vi "grabberpidinit.vi"(9 "setpoint":dbl format="%.2f", 11 "reinitialize? (F) 2":bool) -> (0 "Done? 2":bool)   [LabVIEW 2013]
uses:
  <vilib>/addons/control/pid/pid.llb/PID (DBL).vi
  <vilib>/addons/control/pid/NI_PID_pid.lvlib
panel:
  in  "adjuster":dbl
  in  "PID Gains for Raising/Lowering":T1={"proportional gain (Kc)"=1.2, "integral time (Ti, min)"=0.011, "derivative time (Td, min)"=0.007} {"derivative time (Td, min)" format="%.3f"; "integral time (Ti, min)" format="%.3f"; "proportional gain (Kc)" format="%.3f"}
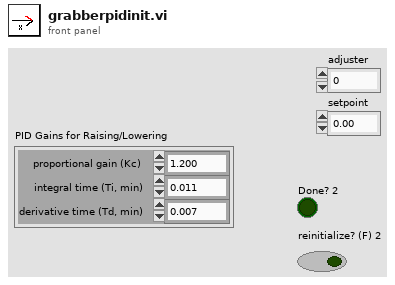
[diagram p1: front panel]
types:
  T1 = cluster{"proportional gain (Kc)":dbl, "integral time (Ti, min)":dbl, "derivative time (Td, min)":dbl}
  T2 = typedef "WPI_EncoderDevRef.ctl" = cluster{"DevStatus":errorcluster, "EncoderIndex":T3, "CounterIndex":T4, "DistancePerCount":dbl, "Decoding Type":T5}
  T3 = typedef "FPGA_EncoderIdx.ctl" = enum8{"Enc 0", "Enc 1", "Enc 2", "Enc 3", "Invalid"}
  T4 = typedef "FPGA_CounterCtrSystemIndex.ctl" = enum8{"Ctr 0", "Ctr 1", "Ctr 2", "Ctr 3", "Ctr 4", "Ctr 5", "Ctr 6", "Ctr 7", "Invalid"}
  T5 = typedef "WPI_EncoderType.ctl" = enum16{"1x", "2x", "4x"}
  T6 = typedef "WPI_MotorControlDeviceRef.ctl" = cluster{"DeviceStatus":errorcluster, "Type":enum16{"PWM", "CAN"}, "PWM":cluster{"Digital Module":T7, "PWM Channel":T8, "DeadBand":T9}, "CAN":cluster{"Device Number":u8, "Control Mode":T10, "Semaphore":T11, "Max Vout":dbl}, "Invert":bool, "TransformRef":T12, "InvTransformRef":T12}
  T7 = typedef "FPGA_TypedefDigitalModule.ctl" = enum16{"Digital Module 1", "Digital Module 2"}
  T8 = typedef "FPGA_DIOPWMChannel.ctl" = enum8{"PWM 1", "PWM 2", "PWM 3", "PWM 4", "PWM 5", "PWM 6", "PWM 7", "PWM 8", "PWM 9", "PWM 10", "Invalid"}
  T9 = typedef "WPI_PWMDeadband.ctl" = cluster{"Name":string, "maxPositivePwm":i32, "minPositivePwm":i32, "centerPwm":i32, "maxNegativePwm":i32, "minNegativePwm":i32, "angularRange":u16}
  T10 = typedef "WPI_CANJaguar_ControlMode.ctl" = enum8{"Percent VBus", "Current", "Speed", "Position", "Voltage"}
  T11 = typedef "Semaphore RefNum" = refnum<k1>
  T12 = typedef "WPI_PWMTransform_ConPane.ctl" = refnum<vi>
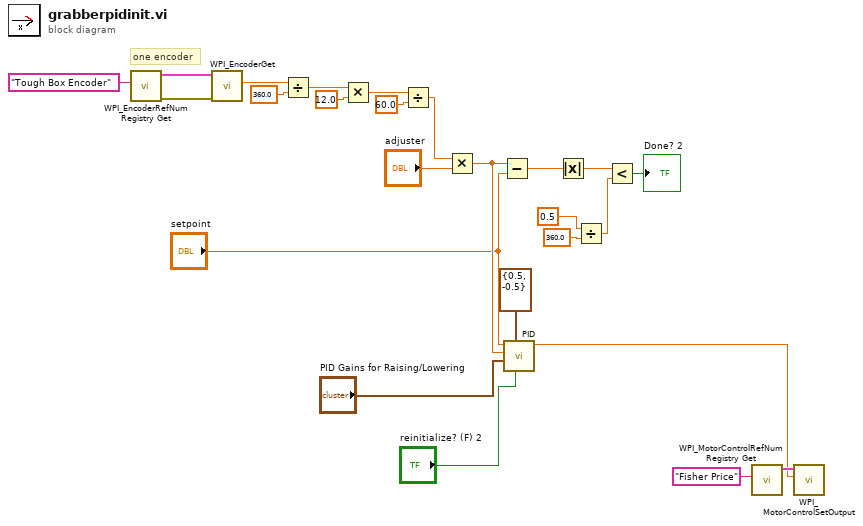
[diagram p0: block diagram]
diagram:
  # "one encoder"
  n1 = call <vilib>:"WPI_EncoderRefNum Registry Get.vi"("refnum name"="Tough Box Encoder") -> ("error out"=w25:errorcluster, "EncoderDevRef"=w24:T2)  [unwired: 9 in]
  n2 = call <vilib>:"WPI_EncoderGet.vi"("error in (no error)"=w25, "EncoderDevRef"=w24) -> ("Distance"=w15:dbl)  [unwired: 4 in, 5 out]
  n3 = Divide(x=w15, y=360.0) -> (x/y=w13:dbl)
  n4 = Multiply(x=w13, y=12.0) -> (x*y=w14:dbl)
  n5 = Divide(x=w14, y=60.0) -> (x/y=w10:dbl)
  n6 = Multiply(x=w10, y="adjuster") -> (x*y=w8:dbl)
  n7 = Subtract(x=w8, y="setpoint") -> (x-y=w20:dbl)
  n8 = call-poly <vilib>:"PID.vi"("reinitialize? (F)"="reinitialize? (F) 2", "output range"=cluster{"output high":dbl, "output low":dbl} {"output high"=0.5, "output low"=-0.5}, "PID gains"="PID Gains for Raising/Lowering", "process variable"=w8, "setpoint"="setpoint") -> ("output"=w1:dbl)  [unwired: 5 in, 1 out]
  n9 = Absolute Value(x=w20) -> (abs(x)=w21:dbl)
  n10 = Divide(x=0.5, y=360.0) -> (x/y=w4:dbl)
  n11 = Less?(x=w21, y=w4) -> (x < y?=→"Done? 2":bool)
  n12 = call <vilib>:"WPI_MotorControlRefNum Registry Get.vi"("refnum name"="Fisher Price") -> ("MotorControlDevRef"=w2:T6)  [unwired: 9 in, 1 out]
  n13 = call <vilib>:"WPI_MotorControlSetOutput.vi"("Output"=w1, "MotorControlDevRef"=w2) -> ()  [unwired: 7 in, 3 out]
